vi "X-Axis Converter v1.00.vi"(4 "Adjust X-Axis Precision":bool, 5 "X-Axis Unit":i32(ring)=1 items=["Point #", "nm", "eV", "meV", "cm-1"], 7 "Old X-Axis Unit":i32(ring)=1 items=["Point #", "nm", "eV", "meV", "cm-1"], 8 "X-Axis input":dbl[](array[numeric])=[500.0, 600.0, 700.0, 800.0, 900.0, 1000.0, 1100.0, 1240.0] format="%.2f") -> (0 "UnitFormatString":string="nm", 1 "X-Axis Output":dbl[](array[numeric]) format="%.4f", 2 "X-Axis Unit String":string, 3 "Precision":i32)   [LabVIEW 2019]
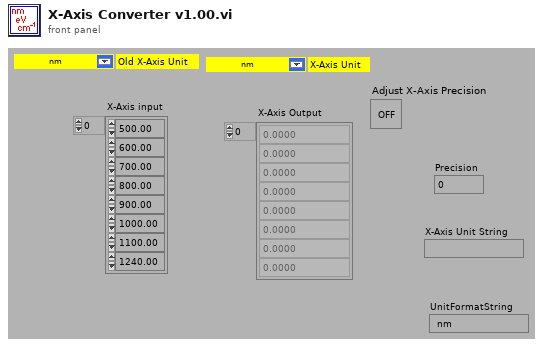
[diagram p1: front panel]
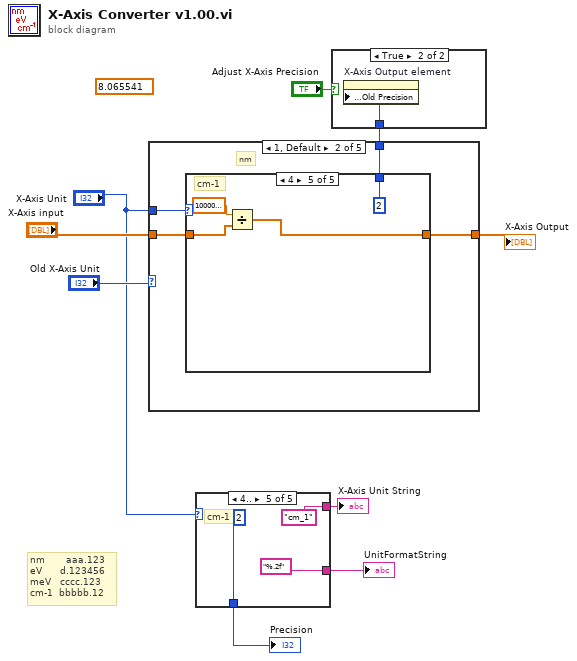
[diagram p0: block diagram]
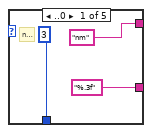
[diagram p2: hidden frame]
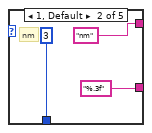
[diagram p3: hidden frame]
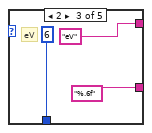
[diagram p4: hidden frame]
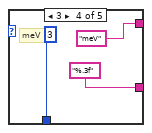
[diagram p5: hidden frame]
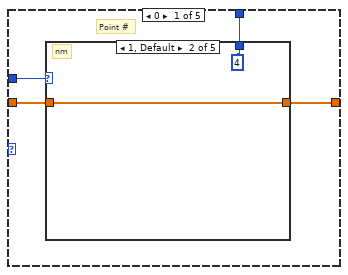
[diagram p7: hidden frame]
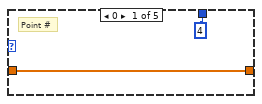
[diagram p8: hidden frame]
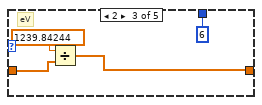
[diagram p9: hidden frame]
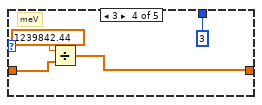
[diagram p10: hidden frame]
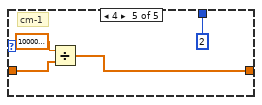
[diagram p11: hidden frame]
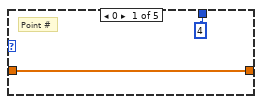
[diagram p12: hidden frame]
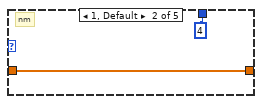
[diagram p13: hidden frame]
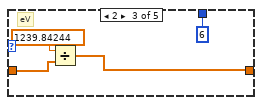
[diagram p14: hidden frame]
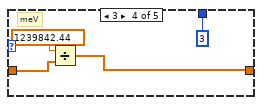
[diagram p15: hidden frame]
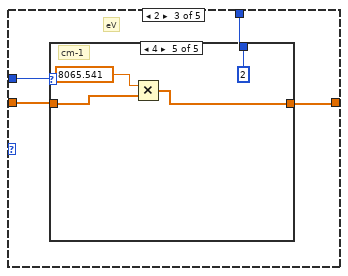
[diagram p16: hidden frame]
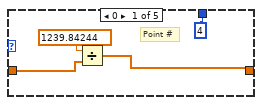
[diagram p17: hidden frame]
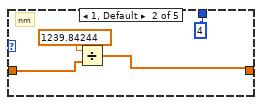
[diagram p18: hidden frame]
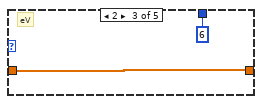
[diagram p19: hidden frame]
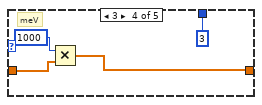
[diagram p20: hidden frame]
diagram:
  (unwired) 8.065541
  # "nm       aaa.123\neV      d.123456\nmeV   cccc.123\ncm-1  bbbbb.12"
  n1 = case shown="1, Default" "Old X-Axis Unit" {
    tunnel: [w12 w32 w51 w73 w95] -> w9
    tunnel: "X-Axis Unit" -> [w11 w31 w53 w75 w97]
    tunnel: [w10 w30 w50 w72 w94] -> w5
    tunnel: "X-Axis input" -> [w13 w33 w52 w74 w96]
    frame 0 {
      # "Point #"
      n2 = case shown="1, Default" w11 {
        tunnel: w13 -> [w14 w17 w20 w24 w28]
        tunnel: [w14 w17 w19 w23 w27] -> w12
        tunnel: [4 4 6 3 2] -> w10
        frame 0 {
          # "Point #"
        }
        frame 1, Default {
          # "nm"
        }
        frame 2 {
          # "eV"
          n3 = Divide(x=1239.84244, y=w20) -> (x/y=w19:dbl[])
        }
        frame 3 {
          # "meV"
          n4 = Divide(x=1239842.44, y=w24) -> (x/y=w23:dbl[])
        }
        frame 4 {
          # "cm-1"
          n5 = Divide(x=10000000.0, y=w28) -> (x/y=w27:dbl[])
        }
      }
    }
    frame 1, Default {
      # "nm"
      n6 = case shown="4" w31 {
        tunnel: w33 -> [w34 w37 w40 w44 w48]
        tunnel: [w34 w37 w39 w43 w47] -> w32
        tunnel: [4 4 6 3 2] -> w30
        frame 0 {
          # "Point #"
        }
        frame 1, Default {
          # "nm"
        }
        frame 2 {
          # "eV"
          n7 = Divide(x=1239.84244, y=w40) -> (x/y=w39:dbl[])
        }
        frame 3 {
          # "meV"
          n8 = Divide(x=1239842.44, y=w44) -> (x/y=w43:dbl[])
        }
        frame 4 {
          # "cm-1"
          n9 = Divide(x=10000000.0, y=w48) -> (x/y=w47:dbl[])
        }
      }
    }
    frame 2 {
      # "eV"
      n10 = case shown="4" w53 {
        tunnel: w52 -> [w55 w59 w62 w66 w71]
        tunnel: [w54 w58 w62 w65 w70] -> w51
        tunnel: [4 4 6 3 2] -> w50
        frame 0 {
          # "Point #"
          n11 = Divide(x=1239.84244, y=w55) -> (x/y=w54:dbl[])
        }
        frame 1, Default {
          # "nm"
          n12 = Divide(x=1239.84244, y=w59) -> (x/y=w58:dbl[])
        }
        frame 2 {
          # "eV"
        }
        frame 3 {
          # "meV"
          n13 = Multiply(x=1000, y=w66) -> (x*y=w65:dbl[])
        }
        frame 4 {
          # "cm-1"
          n14 = Multiply(x=8065.541, y=w71) -> (x*y=w70:dbl[])
        }
      }
    }
    frame 3 {
      # "meV"
      n15 = case shown="4" w75 {
        tunnel: w74 -> [w77 w81 w85 w88 w93]
        tunnel: [w76 w80 w84 w88 w92] -> w73
        tunnel: [4 4 6 3 2] -> w72
        frame 0 {
          # "Point #"
          n16 = Divide(x=1239842.44, y=w77) -> (x/y=w76:dbl[])
        }
        frame 1, Default {
          # "nm"
          n17 = Divide(x=1239842.44, y=w81) -> (x/y=w80:dbl[])
        }
        frame 2 {
          # "eV"
          n18 = Multiply(x=0.001, y=w85) -> (x*y=w84:dbl[])
        }
        frame 3 {
          # "meV"
        }
        frame 4 {
          # "cm-1"
          n19 = Multiply(x=8.065541, y=w93) -> (x*y=w92:dbl[])
        }
      }
    }
    frame 4 {
      # "cm-1"
      n20 = case shown="4" w97 {
        tunnel: w96 -> [w99 w103 w107 w111 w114]
        tunnel: [w98 w102 w106 w112 w114] -> w95
        tunnel: [4 4 6 3 2] -> w94
        frame 0 {
          # "Point #"
          n21 = Divide(x=10000000.0, y=w99) -> (x/y=w98:dbl[])
        }
        frame 1, Default {
          # "nm"
          n22 = Divide(x=10000000.0, y=w103) -> (x/y=w102:dbl[])
        }
        frame 2 {
          # "eV"
          n23 = Divide(x=w107, y=8065.541) -> (x/y=w106:dbl[])
        }
        frame 3 {
          # "meV"
          n24 = Divide(x=w111, y=8.065541) -> (x/y=w112:dbl[])
        }
        frame 4 {
          # "cm-1"
        }
      }
    }
  }
  "X-Axis Output" <- w9
  n25 = case shown="4.." "X-Axis Unit" {
    tunnel: [3 3 6 3 2] -> w3
    tunnel: ["nm" "nm" "eV" "meV" "cm_1"] -> w2
    tunnel: ["%.3f" "%.3f" "%.6f" "%.3f" "%.2f"] -> w1
    frame ..0 {
      # "nm"
    }
    frame 1, Default {
      # "nm"
    }
    frame 2 {
      # "eV"
    }
    frame 3 {
      # "meV"
    }
    frame 4.. {
      # "cm-1"
    }
  }
  "Precision" <- w3
  "X-Axis Unit String" <- w2
  "UnitFormatString" <- w1
  n26 = case shown="True" "Adjust X-Axis Precision" {
    tunnel: w5 -> [_ w131]
    frame False {
    }
    frame True {
      n27 = property on="X-Axis Output element" class="DigNum (strict)"("Old Format & Precision:Old Precision"=w131) -> ()  [unwired: 2 in, 2 out]
    }
  }
